vi "Insert Bound View.vi"(8 "error in (no error)":errorcluster, 9 "Value Publication Time":timestamp, 10 "Selector Value":string, 11 "BoundViewManager in":refnum<class "BoundViewManager.lvclass">) -> (0 "error out":errorcluster, 3 "BoundViewManager out":refnum<class "BoundViewManager.lvclass">)   [LabVIEW 2015, in "BoundViewManager.lvlib" / "BoundViewManager.lvclass"]
uses:
  BoundViewManager.lvclass
  BoundViewManager.lvclass/BoundViewManager.ctl
  Framework/IViewManager/IViewManager/IViewManager.lvclass/IViewManager.ctl
  Framework/IViewable/IViewable Messages/Insert Front Panel Msg/Insert Front Panel Msg.lvclass/Insert Front Panel Msg.ctl
  <vilib>/ActorFramework/Message Enqueuer/Message Enqueuer.lvclass/Message Enqueuer.ctl
  <vilib>/ActorFramework/Message Enqueuer/Message Enqueuer.lvclass
  <vilib>/ActorFramework/Message Enqueuer/Enqueue.vi
  <vilib>/ActorFramework/Message Priority Queue/Priority Enqueue.vi
  Framework/IViewable/IViewable Messages/Insert Front Panel Msg/Insert Front Panel Msg.lvclass
  <vilib>/Composed Systems/Current Value Table/CurrentValueTable.lvclass
  Framework/IViewManager/IViewManager/IViewManager.lvclass
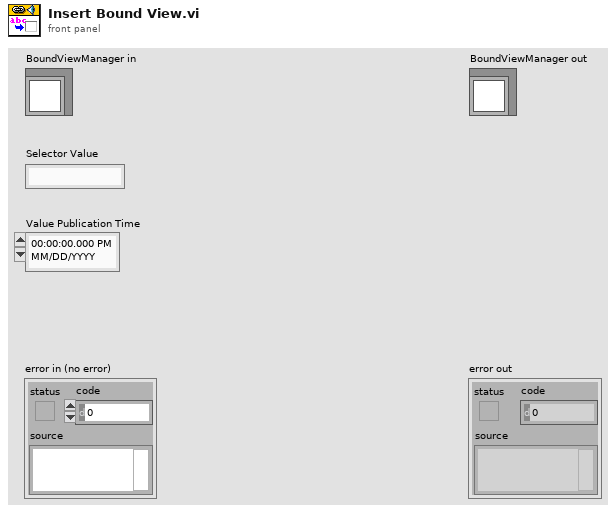
[diagram p1: front panel]
types:
  T1 = typedef "CurrentValueTable.lvlib/CurrentValueTable.lvclass/CurrentValueTable Reference.ctl" = refnum<data-value>
  T2 = typedef "IViewable.lvlib/ProtectedSubpanel.lvclass/Protected Subpanel Reference.ctl" = refnum<data-value>
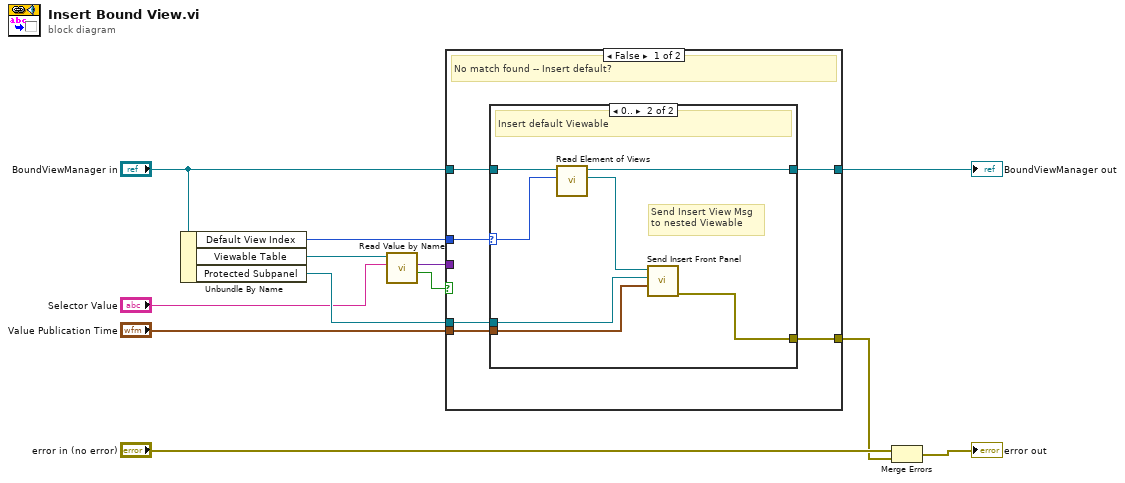
[diagram p0: block diagram]
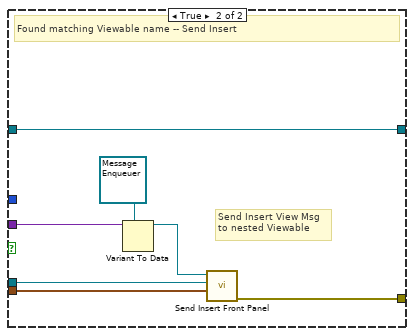
[diagram p3: hidden frame]
diagram:
  n1 = Unbundle By Name("BoundViewManager in") -> ("Default View Index"=w2:i32, "Viewable Table"=w11:T1, "Protected Subpanel"=w10:T2)
  n2 = call <vilib>:"Read Value by Name.vi"("Data Name"="Selector Value", "Current Value Table"=w11) -> ("Value Found?"=w7:bool, "Current Value"=w9:variant)  [unwired: 6 in, 2 out]
  n3 = case shown="False" w7 {
    tunnel: w10 -> [w15 w33]
    tunnel: w9 -> [_ w32]
    tunnel: "Value Publication Time" -> [w14 w29]
    tunnel: [w13 w28] -> w5
    tunnel: "BoundViewManager in" -> [w18 w27]
    tunnel: [w17 w27] -> w3
    tunnel: w2 -> [w16 _]
    frame False {
      # "No match found -- Insert default?"
      n4 = case shown="0.." w16 {
        selector: w16 -> [_ w23]
        tunnel: w18 -> [w19 w26]
        tunnel: [w19 w25] -> w17
        tunnel: w15 -> [_ w22]
        tunnel: w14 -> [_ w21]
        tunnel: [_ w20] -> w13
        frame ..-1 {
          # "No default -- No change"
        }
        frame 0.. {
          # "Send Insert View Msg\nto nested Viewable"
          # "Insert default Viewable"
          n5 = call "Read Element of Views.vi"("Index"=w23, "IViewManager In"=w26) -> ("View Ref"=w24:refnum<class "Message Enqueuer.lvclass">, "IViewManager Out"=w25:refnum<class "BoundViewManager.lvclass">)  [unwired: 7 in, 1 out]
          n6 = call "Send Insert Front Panel.vi"("Request Time"=w21, "Protected Subpanel"=w22, "Message Enqueuer"=w24) -> ("error out"=w20:errorcluster)  [unwired: 7 in, 1 out]
        }
      }
    }
    frame True {
      # "Send Insert View Msg\nto nested Viewable"
      # "Found matching Viewable name -- Send Insert"
      n7 = Variant To Data(type=refnum<class "Message Enqueuer.lvclass"> refnum ("Message Enqueuer"), Variant=w32) -> (data=w30:refnum<class "Message Enqueuer.lvclass">)  [unwired: 1 in, 1 out]
      n8 = call "Send Insert Front Panel.vi"("Request Time"=w29, "Protected Subpanel"=w33, "Message Enqueuer"=w30) -> ("error out"=w28:errorcluster)  [unwired: 7 in, 1 out]
    }
  }
  "BoundViewManager out" <- w3
  n9 = Merge Errors("error in (no error)", w5) -> (→"error out":errorcluster)
